vi "Height SetPoints.vi"(5 "Teleop Local Data In":T1 {"Vision"."Theta_Y" format="%.1f"; "Vision"."Theta_X" format="%.1f"; "Potentio" format="%.1f"; "Drive_Enc_R" format="%.1f"; "Drive_Enc_L" format="%.1f"; "Gyro_Angle" format="%.1f"; "Encoder_Lift" format="%.1f"; "Motor_Lift" format="%.3f"; "Motor_Intake" format="%.3f"; "Drive_Twist" format="%.3f"; "Drive_Forward" format="%.3f"}, 11 "Manual Drive Input":dbl) -> (8 "Set Point out":dbl)   [LabVIEW 2018]
uses:
  Typedefs/typedef_cluster_TeleOp_Local_Data.ctl
  Typedefs/typedef_cluster_Joystick.ctl
  Typedefs/typedef_cluster_Vision.ctl
panel:
  in  "Hatch Low Goal Set Point in":dbl=450.0
  in  "Hatch Middle Goal Set Point":dbl=1100.0
  in  "Hatch Top Goal SetPoint":dbl=2150.0
  in  "Ball Low Goal Set Point in":dbl=750.0
  in  "Ball Middle Goal Set Point":dbl=1400.0
  in  "Ball Top Goal SetPoint":dbl=2450.0
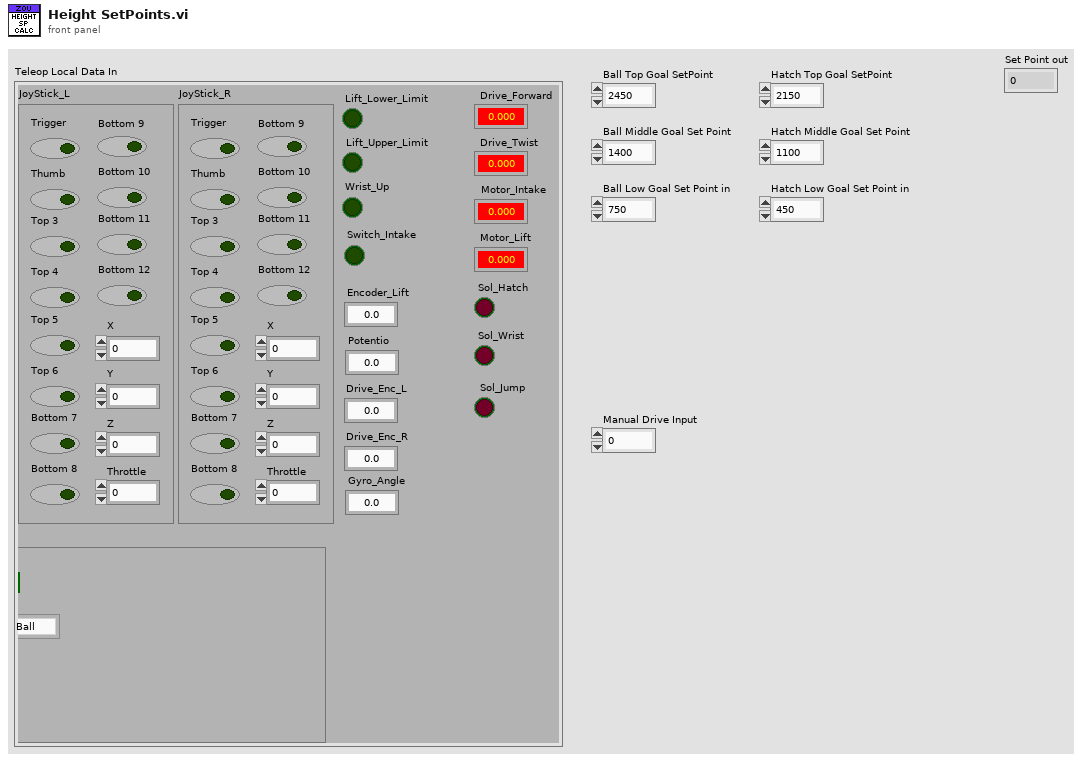
[diagram p1: front panel]
types:
  T1 = typedef "typedef_cluster_TeleOp_Local_Data.ctl" = cluster{"Lift_Lower_Limit":bool, "Wrist_Up":bool, "Switch_Intake":bool, "Encoder_Lift":dbl, "Sol_Wrist":bool, "Motor_Intake":dbl, "Motor_Lift":dbl, "Drive_Forward":dbl, "Drive_Twist":dbl, "Sol_Hatch":bool, "Gyro_Angle":dbl, "Drive_Enc_L":dbl, "Drive_Enc_R":dbl, "JoyStick_L":T2, "JoyStick_R":T2, "Potentio":dbl, "Vision":T3, "Lift_Upper_Limit":bool, "Sol_Jump":bool}
  T2 = typedef "typedef_cluster_Joystick.ctl" = cluster{"X":dbl, "Y":dbl, "Z":dbl, "Throttle":dbl, "Trigger":bool, "Thumb":bool, "Top 3":bool, "Top 4":bool, "Top 5":bool, "Top 6":bool, "Bottom 7":bool, "Bottom 8":bool, "Bottom 9":bool, "Bottom 10":bool, "Bottom 11":bool, "Bottom 12":bool}
  T3 = typedef "typedef_cluster_Vision.ctl" = cluster{"Theta_X":dbl, "Theta_Y":dbl, "Has_Target":bool, "Seek_Ball":bool, "Pipeline":enum16{"Ball", "Dual_Target", "Single_Target"}}
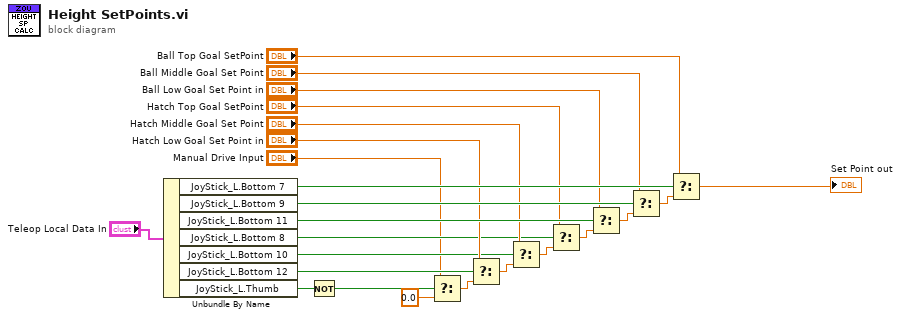
[diagram p0: block diagram]
diagram:
  n1 = Unbundle By Name("Teleop Local Data In") -> ("JoyStick_L.Bottom 7"=w21:bool, "JoyStick_L.Bottom 9"=w22:bool, "JoyStick_L.Bottom 11"=w23:bool, "JoyStick_L.Bottom 8"=w8:bool, "JoyStick_L.Bottom 10"=w7:bool, "JoyStick_L.Bottom 12"=w6:bool, "JoyStick_L.Thumb"=w3:bool)
  n2 = Not(x=w3) -> (.not. x?=w2:bool)
  n3 = Select(t="Manual Drive Input", s=w2, f=0.0 ("t")) -> (s? t:f=w5:dbl)
  n4 = Select(t="Hatch Low Goal Set Point in", s=w6, f=w5) -> (s? t:f=w16:dbl)
  n5 = Select(t="Hatch Middle Goal Set Point", s=w7, f=w16) -> (s? t:f=w17:dbl)
  n6 = Select(t="Hatch Top Goal SetPoint", s=w8, f=w17) -> (s? t:f=w9:dbl)
  n7 = Select(t="Ball Low Goal Set Point in", s=w23, f=w9) -> (s? t:f=w12:dbl)
  n8 = Select(t="Ball Middle Goal Set Point", s=w22, f=w12) -> (s? t:f=w11:dbl)
  n9 = Select(t="Ball Top Goal SetPoint", s=w21, f=w11) -> (s? t:f=→"Set Point out":dbl)
